vi "Check Credential.vi"(8 "error in (no error)":errorcluster, 10 "Credential":T1, 11 "DB in":refnum<class "DB.lvclass">) -> (0 "error out":errorcluster, 2 "Match?":bool, 3 "DB out":refnum<class "DB.lvclass">)   [LabVIEW 2016, in "Database.lvlib" / "DB.lvclass"]
uses:
  DB.lvclass
  Credential.ctl
  Database.lvlib
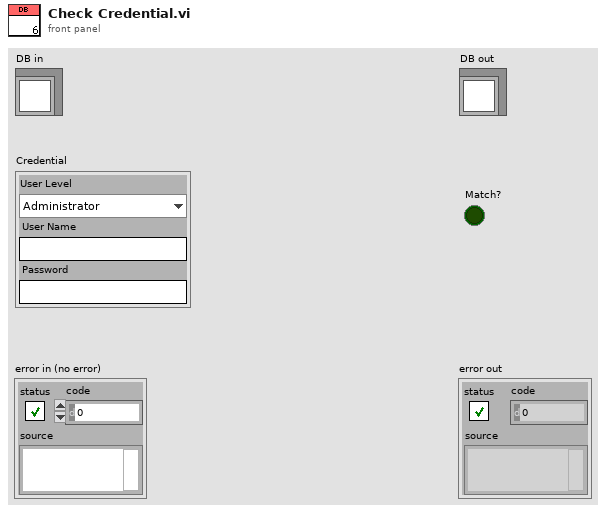
[diagram p1: front panel]
types:
  T1 = typedef "Database.lvlib/Credential.ctl" = cluster{"User Level":enum16{"Administrator", "Engineer", "Operator"}, "User Name":string, "Password":string}
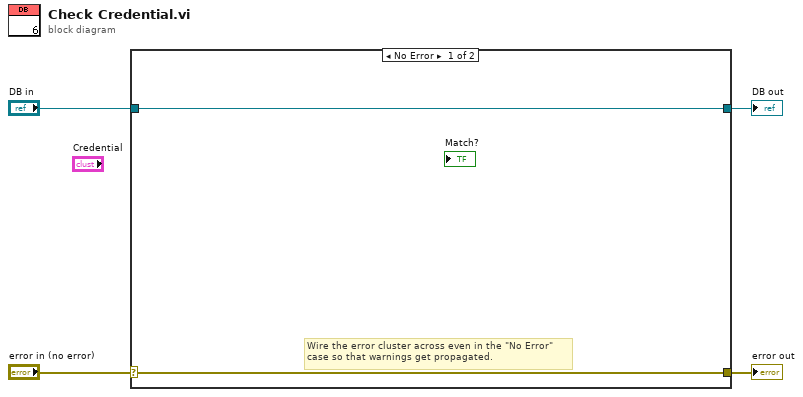
[diagram p0: block diagram]
diagram:
  n1 = case shown="No Error" "error in (no error)" {
    selector: "error in (no error)" -> [w5 w8]
    tunnel: [w5 w8] -> w3
    tunnel: [w6 w7] -> w1
    tunnel: "DB in" -> [w6 w7]
    frame No Error {
      # "Wire the error cluster across even in the \"No Error\"\ncase so that warnings get propagated."
    }
    frame Error {
    }
  }
  "error out" <- w3
  "DB out" <- w1
